vi "SpaceMouse_main.vi"   [LabVIEW 2013]
uses:
  Controls/SpaceMouse_RawInput.ctl
  Controls/SpaceMouse_FilteredInput.ctl
  Controls/SpaceMouse_Buttons.ctl
  Controls/SpaceMouse_Parameters.ctl
  <vilib>/Utility/inputDevices.llb/closeJoystick.vi
  <vilib>/Utility/inputDevices.llb/joystickAcquire.vi
types:
  T1 = typedef "SpaceMouse_Buttons.ctl" = cluster{"Idle":bool, "Button Right":bool, "Button Left":bool}
  T2 = typedef "SpaceMouse_FilteredInput.ctl" = cluster{"X":dbl, "Y":dbl, "Z":dbl, "phi":dbl, "theta":dbl, "psi":dbl}
  T3 = typedef "SpaceMouse_RawInput.ctl" = cluster{"X":i32, "Y":i32, "Z":i32, "phi":i32, "theta":i32, "psi":i32}
  T4 = cluster{"X axis":i32, "Y axis":i32, "Z axis":i32, "X axis rotation":i32, "Y axis rotation":i32, "Z axis rotation":i32, "U axis":i32, "V axis":i32}
  T5 = cluster{"button 1":bool, "button 2":bool, "button 3":bool, "button 4":bool, "button 5":bool, "button 6":bool, "button 7":bool, "button 8":bool, "button 9":bool, "button 10":bool, "button 11":bool, "button 12":bool, "button 13":bool, "button 14":bool, "button 15":bool, "button 16":bool, "button 17":bool, "button 18":bool, "button 19":bool, "button 20":bool, "button 21":bool, "button 22":bool, "button 23":bool, "button 24":bool, "button 25":bool, "button 26":bool, "button 27":bool, "button 28":bool, "button 29":bool, "button 30":bool, "button 31":bool, "button 32":bool}
  T6 = cluster{"X":bool, "Y":bool, "Z":bool, "phi":bool, "theta":bool, "psi":bool}
  T7 = typedef "SpaceMouse_Parameters.ctl" = cluster{"Lowpass Filter Cutoff Frequency":dbl, "Idle Threshold":dbl, "Deadzone":dbl, "Filter Sample Size":i32, "FilterOff":bool, "IntegratorOff":bool}
  T8 = cluster{"[0]":dbl, "[1]":dbl, "[2]":dbl, "[3]":dbl, "[4]":dbl, "[5]":dbl}
  T9 = cluster{"[0]":bool, "[1]":bool, "[2]":bool, "[3]":bool, "[4]":bool, "[5]":bool}
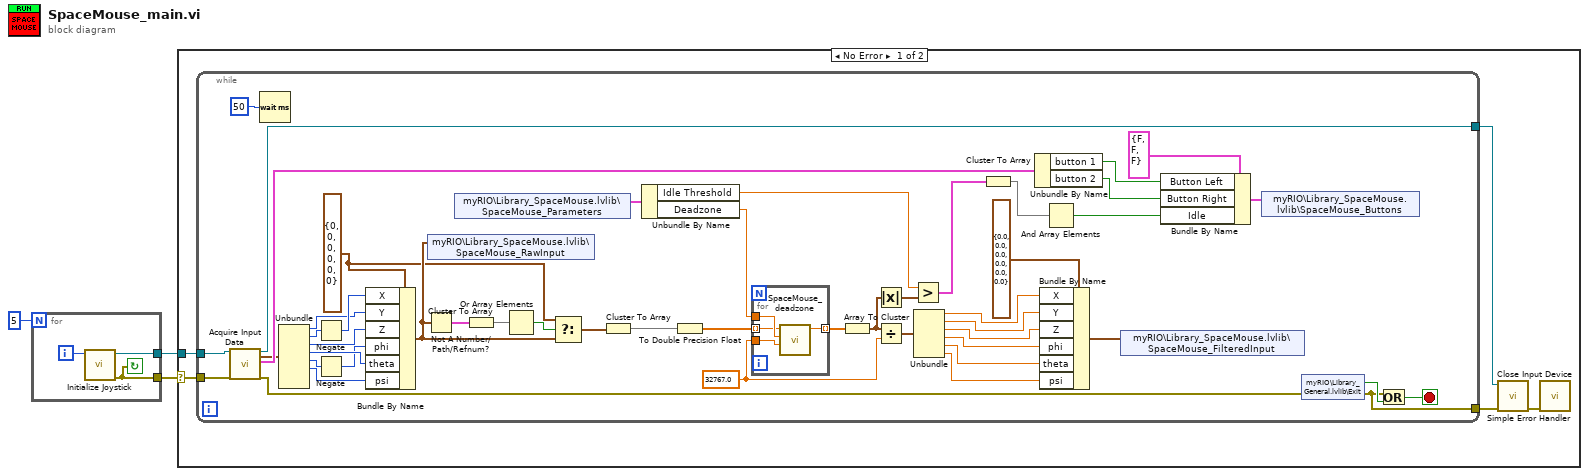
[diagram p0: block diagram]
diagram:
  n1 = for {
    N: 5 -> [_]
    tunnel: [w4] -> w1
    tunnel: [w6] -> w2
    i -> [w5]
    stop <- w4 continue-if-true
    n2 = call <vilib>:"Initialize Joystick.vi"("device index"=w5) -> ("error out"=w4:errorcluster, "device ID"=w6:refnum<k1>)  [unwired: 9 in]
  }
  n3 = case shown="No Error" w1 {
    selector: w1 -> [w8 _]
    tunnel: w2 -> [w9 _]
    frame No Error {
      n4 = while {
        tunnel: [w30] -> w11
        tunnel: [w60] -> w10
        tunnel: w8 -> [w59]
        tunnel: w9 -> [w58]
        stop <- w44 stop-if-true
        w31 = T3 {"X"=0, "Y"=0, "Z"=0, "phi"=0, "theta"=0, "psi"=0} ("SpaceMouse_RawInput")
        w28 = 32767.0
        n5 = call-poly <vilib>:"Acquire Input Data.vi"("device ID"=w58, "error in (no error)"=w59) -> ("device ID"=w60:refnum<k1>, "axis info"=w34:T4, "button info"=w57:T5, "error out"=w27:errorcluster)  [unwired: 13 in, 1 out]
        n6 = Wait (ms)(milliseconds to wait=u32 50 ("Loop wait time (dt)")) -> ()  [unwired: 1 out]
        n7 = Unbundle(w34) -> ("X axis"=w53:i32, "Y axis"=w55:i32, "Z axis"=w52:i32, "X axis rotation"=w51:i32, "Y axis rotation"=w48:i32, "Z axis rotation"=w50:i32)  [unwired: 2 out]
        n8 = Negate(x=w55) -> (-x=w54:i32)
        n9 = Negate(x=w48) -> (-x=w49:i32)
        n10 = Bundle By Name(cluster=w31, "X"=w54, "Y"=w53, "Z"=w52, "phi"=w49, "theta"=w51, "psi"=w50) -> (w32:T3)
        n11 = Not A Number/Path/Refnum?(number/path/refnum=w32) -> (NaN/Path/Refnum?=w36:T6)
        n12 = shared-variable "myRIO\\Library_SpaceMouse.lvlib\\SpaceMouse_RawInput"(w32) -> ()  [unwired: 1 in, 1 out]
        n13 = shared-variable "myRIO\\Library_SpaceMouse.lvlib\\SpaceMouse_Parameters"() -> (w39:T7)  [unwired: 1 in, 1 out]
        n14 = Cluster To Array(cluster=w36) -> (array=w35:bool[])
        n15 = Or Array Elements(Boolean array=w35) -> (logical OR=w12:bool)
        n16 = Select(t=w31, s=w12, f=w32) -> (s? t:f=w33:T3)
        n17 = Cluster To Array(cluster=w33) -> (array=w25:i32[])
        n18 = Unbundle By Name(w39) -> ("Idle Threshold"=w38:dbl, "Deadzone"=w29:dbl)
        n19 = To Double Precision Float(number=w25) -> (double precision float=w13:dbl[])
        n20 = for {
          tunnel: w29 -> [w64]
          tunnel: w28 -> [w63]
          tunnel: w13 -> [w62] mode=indexing
          tunnel: [w61] -> w24 mode=indexing
          n21 = call "SpaceMouse_deadzone.vi"("Space Mouse Input Max"=w63, "Deadzone"=w64, "Filtered Signal"=w62) -> ("Deadzoned & Filtered Signal"=w61:dbl)  [unwired: 8 in]
        }
        n22 = Array To Cluster(array=w24) -> (cluster=w16:T8)
        n23 = Absolute Value(x=w16) -> (abs(x)=w56:T8)
        n24 = Divide(x=w16, y=w28) -> (x/y=w23:T8)
        n25 = Greater?(x=w38, y=w56) -> (0:w26:T9)
        n26 = Unbundle(w23) -> ("[0]"=w22:dbl, "[1]"=w21:dbl, "[2]"=w20:dbl, "[3]"=w19:dbl, "[4]"=w18:dbl, "[5]"=w17:dbl)
        n27 = Cluster To Array(cluster=w26) -> (array=w15:bool[])
        n28 = Unbundle By Name(w57) -> ("button 1"=w46:bool, "button 2"=w45:bool)
        n29 = Bundle By Name(cluster=T2 {"X"=0.0, "Y"=0.0, "Z"=0.0, "phi"=0.0, "theta"=0.0, "psi"=0.0} ("SpaceMouse_FilteredInput"), "X"=w22, "Y"=w21, "Z"=w20, "phi"=w19, "theta"=w18, "psi"=w17) -> (w37:T2)
        n30 = And Array Elements(Boolean array=w15) -> (logical AND=w14:bool)
        n31 = shared-variable "myRIO\\Library_SpaceMouse.lvlib\\SpaceMouse_FilteredInput"(w37) -> ()  [unwired: 1 in, 1 out]
        n32 = Bundle By Name(cluster=T1 {"Idle"=FALSE, "Button Right"=FALSE, "Button Left"=FALSE} ("SpaceMouse_Buttons"), "Button Left"=w46, "Button Right"=w45, "Idle"=w14) -> (w40:T1)
        n33 = shared-variable "myRIO\\Library_SpaceMouse.lvlib\\SpaceMouse_Buttons"(w40) -> ()  [unwired: 1 in, 1 out]
        n34 = shared-variable "myRIO\\Library_General.lvlib\\Exit"(error in=w27) -> (w43:bool, error out=w30:errorcluster)
        n35 = Or(x=w30, y=w43) -> (x .or. y?=w44:bool)
      }
      n36 = call-poly <vilib>:"Close Input Device.vi"("error in (no error)"=w11, "device ID"=w10) -> ("error out"=w7:errorcluster)  [unwired: 8 in]
      n37 = call <vilib>:"Simple Error Handler.vi"("error in (no error)"=w7) -> ()  [unwired: 4 in, 5 out]
    }
    frame Error {
    }
  }
